vi "AuMT8852B Self-Test Results Query.vi"(7 "Action (Return existing results)":T1(ring)=enum."Return existing results", 8 "error in (no error)":errorcluster, 11 "VISA session":refnum<visa-resource-name>) -> (0 "error out":errorcluster, 2 "error code":i32, 3 "VISA session out":refnum<visa-resource-name>, 4 "Results":string)   [LabVIEW 2017]
doc: "Anritsu MT8852B Bluetooth Tester\n\nReturns detailed self-test results.\n\nINPUTS\nAction - whether to return the results of a new test or the results of the previous test.\n\nOUTPUTS\nResults - the individual pass/fail result of each test."
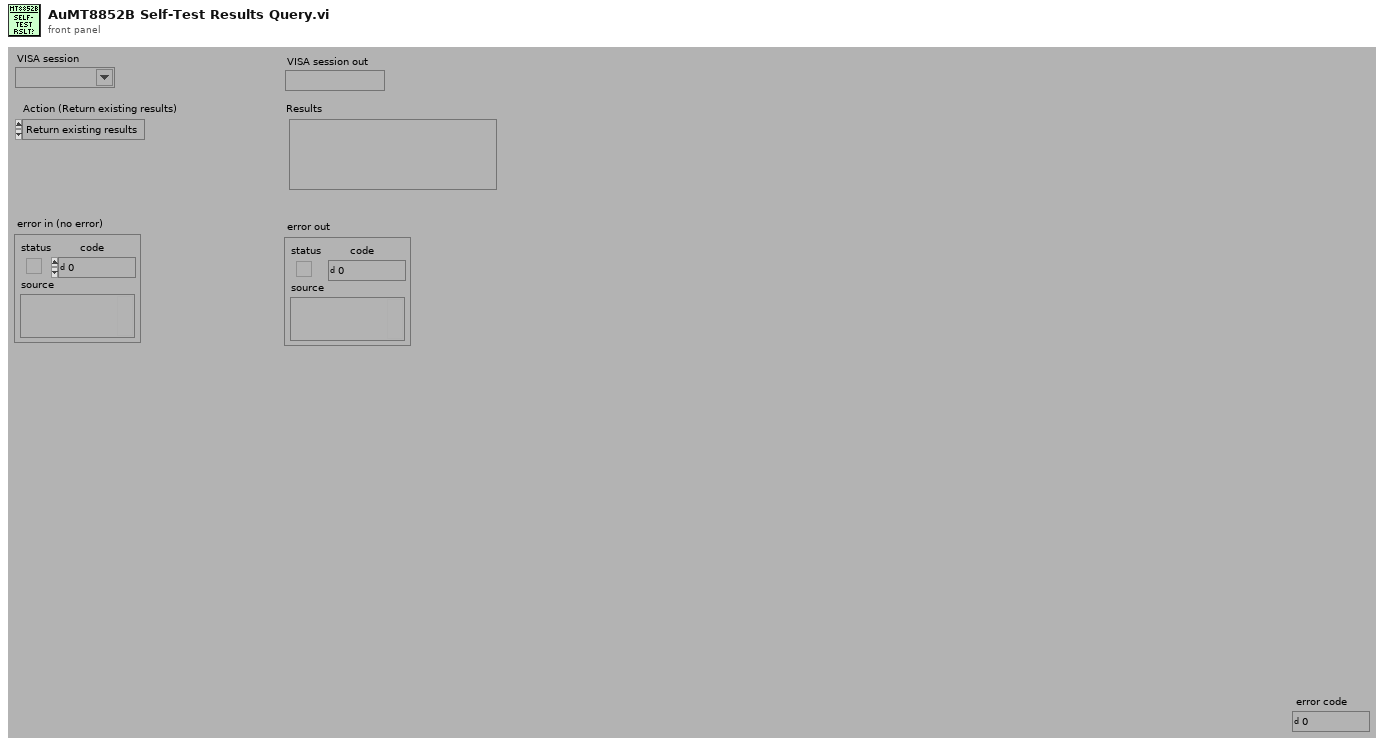
[diagram p1: front panel]
types:
  T1 = enum16{"Execute new test", "Return existing results"}
  T2 = enum16{"Simulate", "Range check", "Cache", "Query instrument status"}
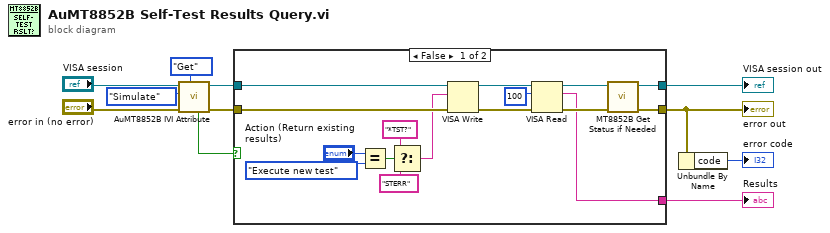
[diagram p0: block diagram]
diagram:
  n1 = call <instrlib>:"AuMT8852B IVI Attribute.vi"("Set/Get (Set)"=enum16{"Set", "Get"}."Get", "error in (no error)"="error in (no error)", "Flag (Simulate)"=T2."Simulate", "VISA session"="VISA session") -> ("error out"=w7:errorcluster, "VISA session out"=w8:refnum<visa-resource-name>, "Value out"=w4:bool)  [unwired: 5 in]
  n2 = case shown="False" w4 {
    tunnel: [w24 w29] -> w2
    tunnel: [w25 w30] -> w9
    tunnel: w8 -> [w27 w30]
    tunnel: w7 -> [w26 w29]
    tunnel: [w12 ""] -> w1
    frame False {
      n3 = Equal?(x="Action (Return existing results)", y=T1."Execute new test") -> (x = y?=w16:bool)
      n4 = Select(t="*TST?", s=w16, f="STERR") -> (s? t:f=w13:string)
      n5 = VISA Write(VISA resource name=w27, write buffer=w13, error in (no error)=w26) -> (VISA resource name out=w23:refnum<visa-resource-name>, error out=w21:errorcluster)  [unwired: 1 out]
      n6 = VISA Read(VISA resource name=w23, byte count=u32 100 ("byte count (0)"), error in (no error)=w21) -> (VISA resource name out=w20:refnum<visa-resource-name>, read buffer=w12:string, error out=w19:errorcluster)  [unwired: 1 out]
      n7 = call <instrlib>:"MT8852B Get Status if Needed.vi"("error in (no error)"=w19, "VISA session"=w20) -> ("error out"=w24:errorcluster, "VISA session out"=w25:refnum<visa-resource-name>)  [unwired: 8 in]
    }
    frame True {
    }
  }
  "error out" <- w2
  "VISA session out" <- w9
  "Results" <- w1
  n8 = Unbundle By Name(w2) -> ("code"=→"error code":i32)
